vi "时间日期字符串至时间标识转换.vi"(11 "时间日期字符串":string="1904/01/01 00:00:00") -> (3 "时间标识":timestamp format="%<%Y/%m/%d\n%H:%M:%S>T")   [LabVIEW 2016, in "数据传输系统-02.lvlib"]
panel:
  out "数组 2":i32[](array[numeric])
  out "数组":string[](array[string])
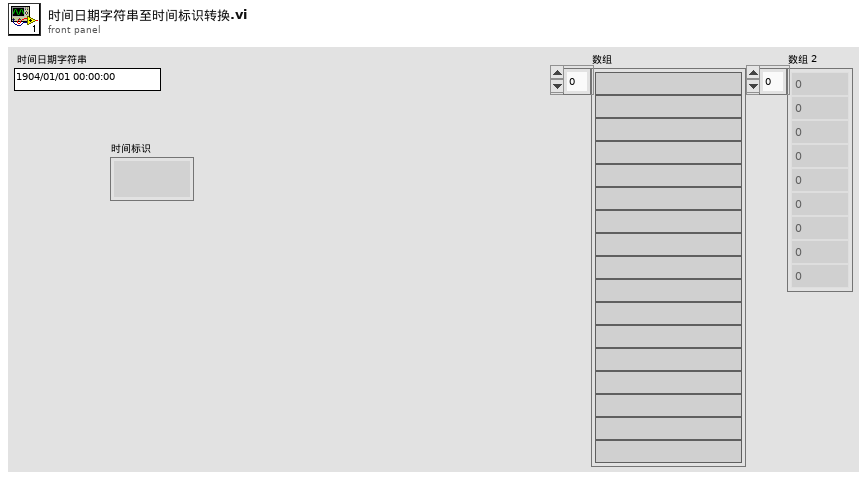
[diagram p1: front panel]
types:
  T1 = typedef "LVDateTimeRec.ctl" = cluster{"秒数的小数部分":dbl, "秒":i32, "分":i32, "时":i32, "日":i32, "月":i32, "年":i32, "天数（周）":i32, "天数（年）":i32, "DST":i32}
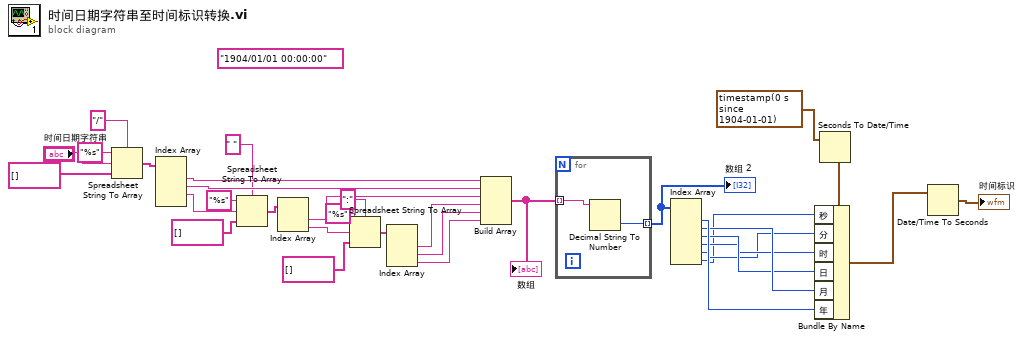
[diagram p0: block diagram]
diagram:
  (unwired) "1904/01/01 00:00:00"
  n1 = Spreadsheet String To Array(delimiter (Tab)="/" ("分隔符(Tab)"), format string="%s" ("格式字符串"), spreadsheet string="时间日期字符串", array type (2D Dbl)=string[] []) -> (array=w26:string[])
  n2 = Index Array(array=w26) -> (element #1=w25:string, element #2=w24:string, element #3=w23:string)  [unwired: 4 in, 1 out]
  n3 = Spreadsheet String To Array(delimiter (Tab)=" " ("分隔符(Tab)"), format string="%s" ("格式字符串"), spreadsheet string=w23, array type (2D Dbl)=string[] []) -> (array=w19:string[])
  n4 = Index Array(array=w19) -> (element #1=w18:string, element #2=w17:string)  [unwired: 2 in]
  n5 = Spreadsheet String To Array(delimiter (Tab)=":" ("分隔符(Tab)"), format string="%s" ("格式字符串"), spreadsheet string=w17, array type (2D Dbl)=string[] []) -> (array=w13:string[])
  n6 = Index Array(array=w13) -> (element #1=w12:string, element #2=w11:string, element #3=w10:string)  [unwired: 3 in]
  n7 = Build Array(w25, w24, w18, w12, w11, w10) -> (w9:string[])
  "数组" <- w9
  n8 = for {
    tunnel: w9 -> [w35] mode=indexing
    tunnel: [w34] -> w8 mode=indexing
    n9 = Decimal String To Number(string=w35) -> (number=w34:i32)  [unwired: 2 in, 1 out]
  }
  "数组 2" <- w8
  n10 = Index Array(array=w8) -> (element #1=w7:i32, element #2=w6:i32, element #3=w5:i32, element #4=w4:i32, element #5=w3:i32, element #6=w2:i32)  [unwired: 6 in]
  n11 = Seconds To Date/Time(time stamp (now)=timestamp(0 s since 1904-01-01) ("时间标识")) -> (date time rec=w32:T1)  [unwired: 1 in]
  n12 = Bundle By Name(cluster=w32, "秒"=w2, "分"=w3, "时"=w4, "日"=w5, "月"=w6, "年"=w7) -> (w31:T1)
  n13 = Date/Time To Seconds(2:w31) -> (0:→"时间标识":timestamp)  [unwired: 1 in]
